vi "BuildTestFromProjectItem.vi"(8 "error in (no error)":errorcluster, 10 "ProjectItem Refnum":refnum<vi>, 11 "TestBuilder in":refnum<class "TestBuilder.lvclass">) -> (0 "error out":errorcluster, 2 "Test":refnum<class "Test.lvclass">, 3 "TestBuilder out":refnum<class "TestBuilder.lvclass">)   [LabVIEW 2019, in "TestBuilder.lvclass"]
doc: "Builds a test from the specified <B>ProjectItem</B>."
uses:
  TestBuilder.lvclass
  Test/Test.lvclass
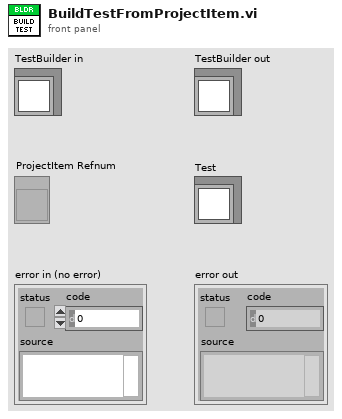
[diagram p1: front panel]
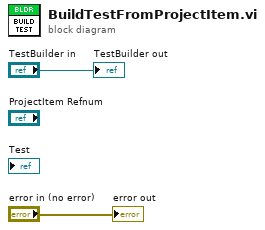
[diagram p0: block diagram]
diagram:
  "error out" <- "error in (no error)"
  "TestBuilder out" <- "TestBuilder in"
